vi "SshClose.vi"(3 "SshStream in":refnum<k24>, 9 "error in (no error)":errorcluster) -> (6 "sortie d'erreur":errorcluster caption="error out")   [LabVIEW 2009]
uses:
  C:/Ohana/LV2009/OhanaOS-LV81/Instruments/Keyword/Controller/Tamir.sharpSsh.dll
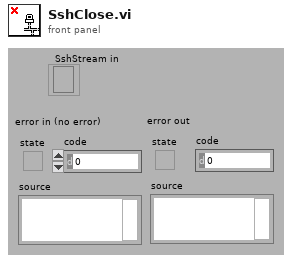
[diagram p1: front panel]
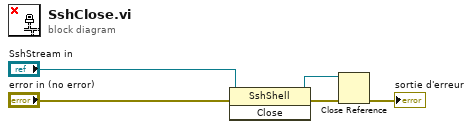
[diagram p0: block diagram]
diagram:
  n1 = invoke class="SshShell" method="Close"(reference="SshStream in", error in="error in (no error)") -> (reference out=w4:refnum<k24>, error out=w3:errorcluster)  [unwired: 1 in, 1 out]
  n2 = Close Reference(reference=w4, error in (no error)=w3) -> (error out=→"sortie d'erreur":errorcluster)
